vi "LibXML_FreeNode.vi"(8 "error in":errorcluster, 11 "node":u32) -> (0 "error out":errorcluster)   [LabVIEW 2019, in "Tools.lvlib" / "LibXML.lvlib"]
doc: "Free a pointer to a node input."
uses:
  LibXML.lvlib
  dll/libxml2.dll
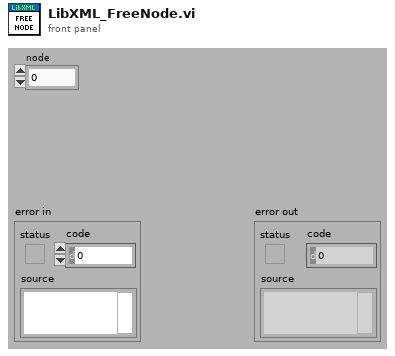
[diagram p1: front panel]
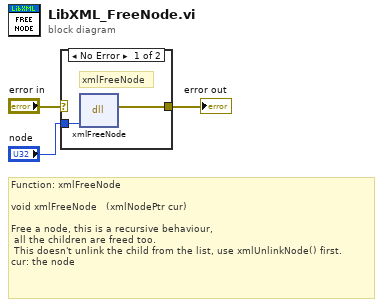
[diagram p0: block diagram]
diagram:
  # "Function: xmlFreeNode\n\nvoid\txmlFreeNode\t\t\t(xmlNodePtr cur)\n\nFree a node, this is a recursive behaviour,\n all the children are freed too.\n This doesn't unlink the child from the list, use xmlUnlinkNode() first.\ncur:\tthe node"
  n1 = case shown="No Error" "error in" {
    selector: "error in" -> [_ w6]
    tunnel: [w5 w6] -> w2
    tunnel: "node" -> [w4 _]
    frame No Error {
      # "xmlFreeNode"
      n2 = dll-call lib="C:/Projects/_Prywatne/MyCIT/Framework/Tools/XML/LibXML/dll/libxml2.dll" fn="xmlFreeNode"("node"=w4) -> (error out=w5:errorcluster)  [unwired: 5 in, 1 out]
    }
    frame Error {
    }
  }
  "error out" <- w2
